vi "SHA-1 (File).vi"(10 "filepath":path) -> (2 "SHA-1 hash":string)   [LabVIEW 2013, in "SHA-1.lvlib"]
uses:
  SHA-1.lvlib
  SHA-1.lvclass
  Data-vector.ctl
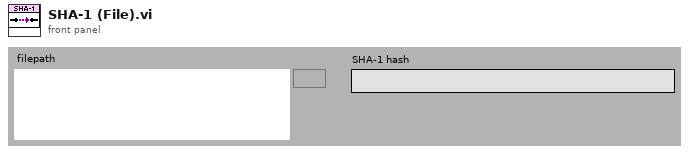
[diagram p1: front panel]
types:
  T1 = typedef "SHA-1.lvlib/SHA-1.lvclass/Data-vector.ctl" = cluster{"Data[ ]":u8[], "end":bool}
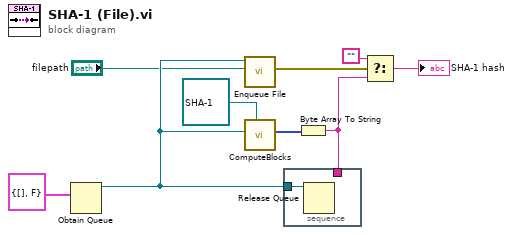
[diagram p0: block diagram]
diagram:
  n1 = Obtain Queue(element data type=T1 {"Data[ ]"=[], "end"=FALSE} ("cluster")) -> (queue out=w3:refnum<queue>)  [unwired: 4 in, 2 out]
  n2 = call "Enqueue File.vi"("filepath"="filepath", "Blocks queue"=w3) -> ("error out"=w1:errorcluster)  [unwired: 9 in]
  n3 = call-dynamic "ComputeBlocks.vi"("SHA-1"=refnum<class "SHA-1.lvclass"> refnum, "blocks queue"=w3) -> ("hash"=w5:u8[])  [unwired: 9 in]
  n4 = Byte Array To String(unsigned byte array=w5) -> (string=w4:string)
  n5 = stacked-sequence {
    tunnel: w3 -> [w10]
    tunnel: w4 -> [_]
    frame #0 {
      n6 = Release Queue(queue=w10) -> ()  [unwired: 2 in, 3 out]
    }
  }
  n7 = Select(t="", s=w1, f=w4) -> (s? t:f=→"SHA-1 hash":string)
